vi "GetStatus.vi"(8 "error in (no error)":errorcluster, 11 "GS in":refnum<class "GuiderSetup.lvclass">) -> (0 "error out":errorcluster, 3 "GS out":refnum<class "GuiderSetup.lvclass">)   [LabVIEW 2018, in "GuiderSetup.lvclass"]
uses:
  GuiderSetup.lvclass
  C:/Users/devstaff/sparc4/s4gui/Versao ZeroMQ REQ-REP/SPARC4_GUI -v1.0.0/S4GUI/S4GUI.lvclass
  S4GUI/S4GUI.lvclass/S4GUI.ctl
  Instrument/Instrument.lvclass/Instrument.ctl
  Device/Optics/Optics.lvclass/Optics.ctl
  Server/Server.lvclass/Server.ctl
  Device/Optics/Opt_Continuous/Opt_Continuous.lvclass
  C:/Users/devstaff/sparc4/s4gui/Versao ZeroMQ REQ-REP/SPARC4_GUI -v1.0.0/Device/Optics/Optics.lvclass
  Instrument/Instrument.lvclass
  C:/Users/devstaff/sparc4/s4gui/Versao ZeroMQ REQ-REP/SPARC4_GUI -v1.0.0/Server/Server.lvclass
  S4GUI/S4GUI.lvclass
  Device/Optics/Optics.lvclass
  Server/Server.lvclass
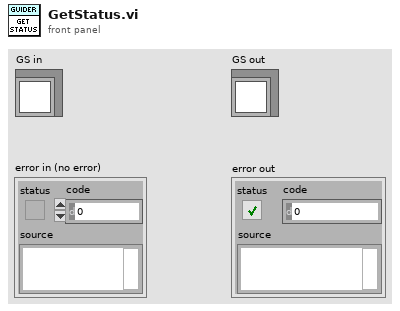
[diagram p1: front panel]
types:
  T1 = cluster{"Trigger Mode Status":string, "String output":string, "Instrument Status":cluster{"WPROT pos":dbl, "WPSEL pos":dbl, "GMIR pos":dbl, "GFOC pos":dbl, "CALW pos":dbl, "ASEL pos":dbl, "mode":bool, "String Status":string, "connection":bool, "operational":bool}, "Sync Box State":i32, "Trigger General Status":string, "Instrument States":cluster{"WPSEL State":i32, "WPROT State":i32, "CALW State":i32, "ASEL State":i32, "GMIR State":i32, "GFOC State":i32}, "Instrument Pos Names":cluster{"WPROT posname":string, "WPSEL posname":string, "CALW posname":string, "ASEL posname":string}, "ChannelA_Status":cluster{"Current exp":dbl, "Frames done":u32, "LastFileImage":string, "CamStatus":string, "Run state":u32, "connection":bool, "Cooler ON/OFF":i16, "Currently temperature":i16, "Temperature Status":string, "target  temp":i16, "conf runing":bool, "FT":bool, "UsedDisk":u16, "operational":bool}, "WPROT seq":u16, "ChannelB_Status":cluster{"Current exp":dbl, "Frames done":u32, "LastFileImage":string, "CamStatus":string, "Run state":u32, "connection":bool, "Cooler ON/OFF":i16, "Currently temperature":i16, "Temperature Status":string, "target  temp":i16, "conf runing":bool, "FT":bool, "UsedDisk":u16, "operational":bool}, "ChannelC_Status":cluster{"Current exp":dbl, "Frames done":u32, "LastFileImage":string, "CamStatus":string, "Run state":u32, "connection":bool, "Cooler ON/OFF":i16, "Currently temperature":i16, "Temperature Status":string, "target  temp":i16, "conf runing":bool, "FT":bool, "UsedDisk":u16, "operational":bool}, "ChannelD_Status":cluster{"Current exp":dbl, "Frames done":u32, "LastFileImage":string, "CamStatus":string, "Run state":u32, "connection":bool, "Cooler ON/OFF":i16, "Currently temperature":i16, "Temperature Status":string, "target  temp":i16, "conf runing":bool, "FT":bool, "UsedDisk":u16, "operational":bool}, "ChannelA_CCD":cluster{"ACQUISITION_MODE":u8, "TRIGGER_MODE":u8, "READ_MODE":u8, "PREAMP":u8, "READOUT_RATE":u8, "VERTICAL_SHIFT_SPEED":u8, "EM_MODE":u8, "EM_GAIN":u16, "SHUTTER_MODE":u8, "SHUTTER_TTL":u8, "SHUTTER_OPENNING_TIME":u16, "SHUTTER_CLOSING_TIME":u16, "VBIN":u16, "HBIN":u16, "INITIAL_LINE":u16, "INITIAL_COLUMN":u16, "FINAL_LINE":u16, "FINAL_COLUMN":u16, "FRAME_TRANSFER":bool, "VERTICAL_CLOCK_VOLTAGE":u8, "AD_CHANNEL":u32}, "ChannelB_CCD ":cluster{"ACQUISITION_MODE":u8, "TRIGGER_MODE":u8, "READ_MODE":u8, "PREAMP":u8, "READOUT_RATE":u8, "VERTICAL_SHIFT_SPEED":u8, "EM_MODE":u8, "EM_GAIN":u16, "SHUTTER_MODE":u8, "SHUTTER_TTL":u8, "SHUTTER_OPENNING_TIME":u16, "SHUTTER_CLOSING_TIME":u16, "VBIN":u16, "HBIN":u16, "INITIAL_LINE":u16, "INITIAL_COLUMN":u16, "FINAL_LINE":u16, "FINAL_COLUMN":u16, "FRAME_TRANSFER":bool, "VERTICAL_CLOCK_VOLTAGE":u8, "AD_CHANNEL":u32}, "ChannelC_CCD":cluster{"ACQUISITION_MODE":u8, "TRIGGER_MODE":u8, "READ_MODE":u8, "PREAMP":u8, "READOUT_RATE":u8, "VERTICAL_SHIFT_SPEED":u8, "EM_MODE":u8, "EM_GAIN":u16, "SHUTTER_MODE":u8, "SHUTTER_TTL":u8, "SHUTTER_OPENNING_TIME":u16, "SHUTTER_CLOSING_TIME":u16, "VBIN":u16, "HBIN":u16, "INITIAL_LINE":u16, "INITIAL_COLUMN":u16, "FINAL_LINE":u16, "FINAL_COLUMN":u16, "FRAME_TRANSFER":bool, "VERTICAL_CLOCK_VOLTAGE":u8, "AD_CHANNEL":u32}, "ChannelD_CCD":cluster{"ACQUISITION_MODE":u8, "TRIGGER_MODE":u8, "READ_MODE":u8, "PREAMP":u8, "READOUT_RATE":u8, "VERTICAL_SHIFT_SPEED":u8, "EM_MODE":u8, "EM_GAIN":u16, "SHUTTER_MODE":u8, "SHUTTER_TTL":u8, "SHUTTER_OPENNING_TIME":u16, "SHUTTER_CLOSING_TIME":u16, "VBIN":u16, "HBIN":u16, "INITIAL_LINE":u16, "INITIAL_COLUMN":u16, "FINAL_LINE":u16, "FINAL_COLUMN":u16, "FRAME_TRANSFER":bool, "VERTICAL_CLOCK_VOLTAGE":u8, "AD_CHANNEL":u32}, "CHA_Checked Params":cluster{"ACQUISITION_MODE":bool, "TRIGGER_MODE":bool, "READ_MODE":bool, "PREAMP":bool, "READOUT_RATE":bool, "VERTICAL_SHIFT_SPEED":bool, "EM_MODE":bool, "EM_GAIN":bool, "SHUTTER_MODE":bool, "SHUTTER_TTL":bool, "SHUTTER_OPENING_TIME":bool, "SHUTTER_CLOSING_TIME":bool, "VBIN":bool, "HBIN":bool, "INITIAL_LINE":bool, "INITIAL_COLUMN":bool, "FINAL_LINE":bool, "FINAL_COLUMN":bool, "FRAME_TRANSFER":bool, "VERTICAL_CLOCK_VOLTAGE":bool, "AD_CHANNEL":bool}, "CHB_Checked Params":cluster{"ACQUISITION_MODE":bool, "TRIGGER_MODE":bool, "READ_MODE":bool, "PREAMP":bool, "READOUT_RATE":bool, "VERTICAL_SHIFT_SPEED":bool, "EM_MODE":bool, "EM_GAIN":bool, "SHUTTER_MODE":bool, "SHUTTER_TTL":bool, "SHUTTER_OPENING_TIME":bool, "SHUTTER_CLOSING_TIME":bool, "VBIN":bool, "HBIN":bool, "INITIAL_LINE":bool, "INITIAL_COLUMN":bool, "FINAL_LINE":bool, "FINAL_COLUMN":bool, "FRAME_TRANSFER":bool, "VERTICAL_CLOCK_VOLTAGE":bool, "AD_CHANNEL":bool}, "CHC_Checked Params":cluster{"ACQUISITION_MODE":bool, "TRIGGER_MODE":bool, "READ_MODE":bool, "PREAMP":bool, "READOUT_RATE":bool, "VERTICAL_SHIFT_SPEED":bool, "EM_MODE":bool, "EM_GAIN":bool, "SHUTTER_MODE":bool, "SHUTTER_TTL":bool, "SHUTTER_OPENING_TIME":bool, "SHUTTER_CLOSING_TIME":bool, "VBIN":bool, "HBIN":bool, "INITIAL_LINE":bool, "INITIAL_COLUMN":bool, "FINAL_LINE":bool, "FINAL_COLUMN":bool, "FRAME_TRANSFER":bool, "VERTICAL_CLOCK_VOLTAGE":bool, "AD_CHANNEL":bool}, "CHD_Checked Params":cluster{"ACQUISITION_MODE":bool, "TRIGGER_MODE":bool, "READ_MODE":bool, "PREAMP":bool, "READOUT_RATE":bool, "VERTICAL_SHIFT_SPEED":bool, "EM_MODE":bool, "EM_GAIN":bool, "SHUTTER_MODE":bool, "SHUTTER_TTL":bool, "SHUTTER_OPENING_TIME":bool, "SHUTTER_CLOSING_TIME":bool, "VBIN":bool, "HBIN":bool, "INITIAL_LINE":bool, "INITIAL_COLUMN":bool, "FINAL_LINE":bool, "FINAL_COLUMN":bool, "FRAME_TRANSFER":bool, "VERTICAL_CLOCK_VOLTAGE":bool, "AD_CHANNEL":bool}, "Trigger_connection":bool, "TCSPD_connection":bool, "TCS extended":string, "TCS id":u32, "S4ICS id":u32, "focus pos":i32, "Focus_connection":bool, "WS_connection":bool, "weather status":cluster{"broker":string, "version":string, "date":string, "hour":string, "outHumidity":string, "inHumidity":string, "inTemp":string, "outTemp":string, "windSpeed":string, "windDirection":string, "pressure":string, "dewOut":string, "dewIn":string, "leaf":string, "rain":string, "windChill":string}, "GS STATUS cluster":cluster{"FocusPhot":dbl, "FocusPolar":dbl, "FocusEffic":dbl, "FocusInstrum":dbl, "ICS":bool, "AG":bool, "BROKER":string}, "TCSPD_operational":bool, "Focus_operational":bool}
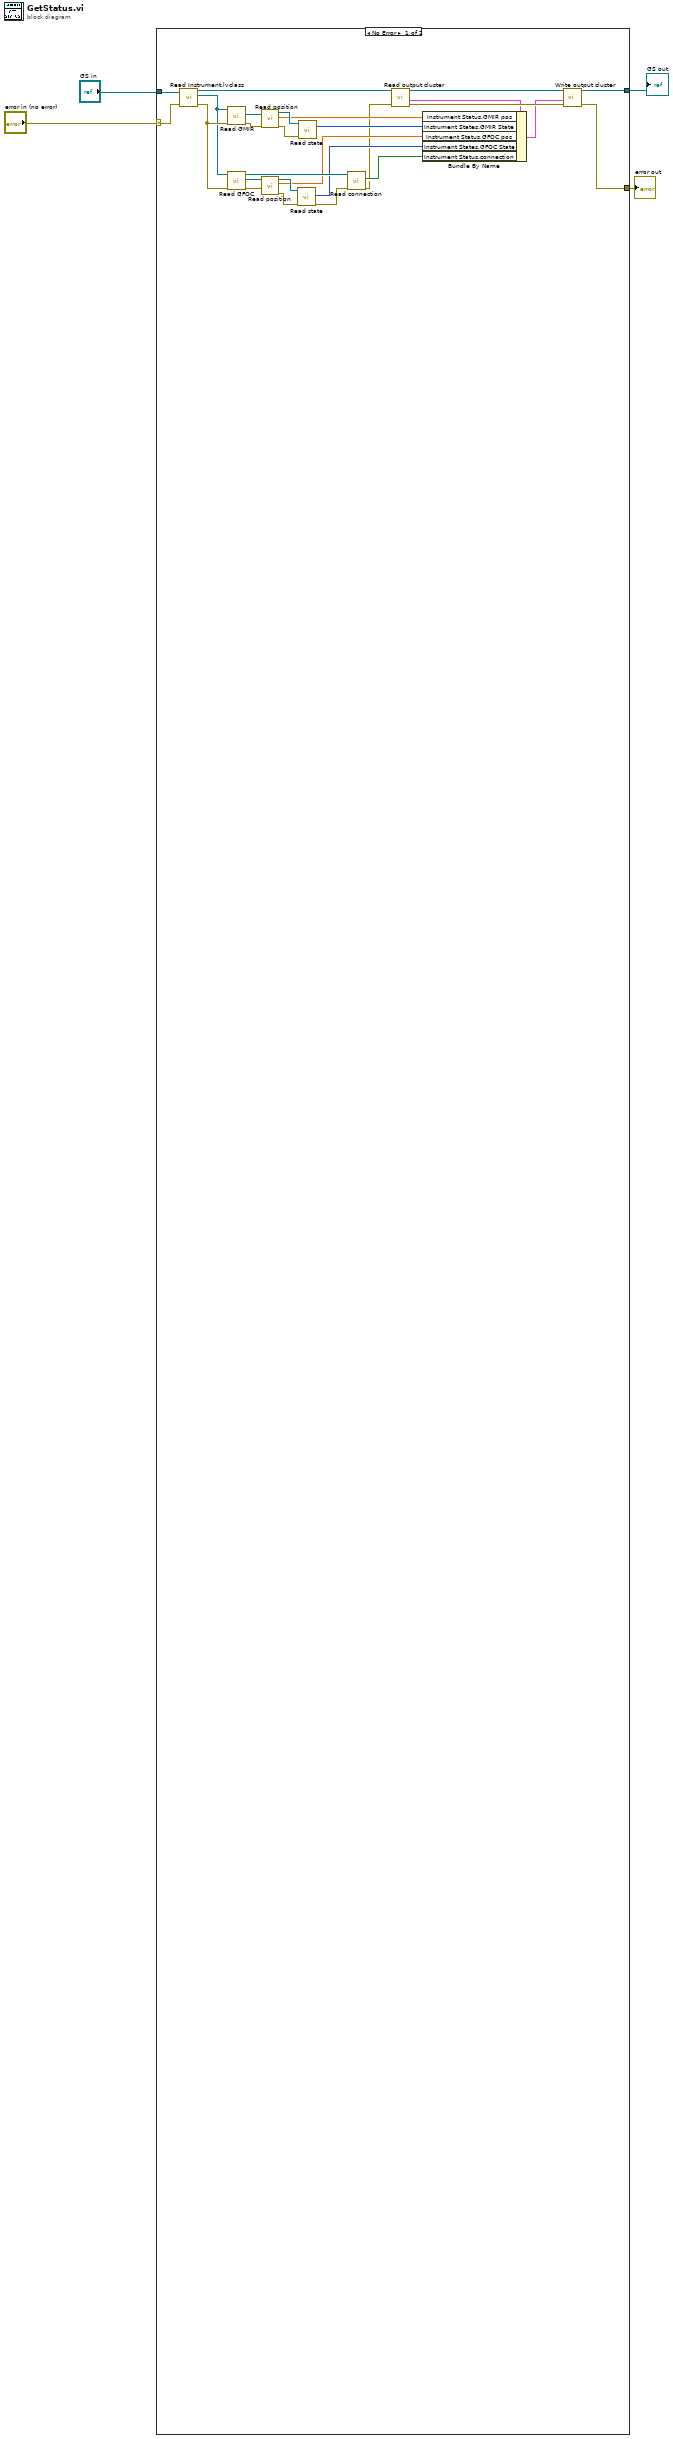
[diagram p0: block diagram]
diagram:
  n1 = case shown="No Error" "error in (no error)" {
    selector: "error in (no error)" -> [w20 w32]
    tunnel: "GS in" -> [w19 w33]
    tunnel: [w12 w33] -> w2
    tunnel: [w11 w32] -> w1
    frame No Error {
      n2 = call "Read Instrument.lvclass.vi"("error in (no error)"=w20, "S4ACS_GUI in"=w19) -> ("error out"=w21:errorcluster, "Instrument.lvclass"=w18:refnum<class "Instrument.lvclass">, "S4ACS_GUI out"=w10:refnum<class "GuiderSetup.lvclass">)  [unwired: 7 in]
      n3 = call "Read GMIR.vi"("error in (no error)"=w21, "Instrument in"=w18) -> ("error out"=w31:errorcluster, "Opt_Continuous.lvclass"=w30:refnum<class "Opt_Continuous.lvclass">)  [unwired: 7 in, 1 out]
      n4 = call "Read GFOC.vi"("error in (no error)"=w21, "Instrument in"=w18) -> ("error out"=w28:errorcluster, "Opt_Continuous.lvclass"=w29:refnum<class "Opt_Continuous.lvclass">, "Instrument out"=w23:refnum<class "Instrument.lvclass">)  [unwired: 7 in]
      n5 = call "Read position.vi"("error in (no error)"=w31, "Optics in"=w30) -> ("error out"=w26:errorcluster, "position"=w16:dbl, "Optics out"=w27:refnum<class "Opt_Continuous.lvclass">)  [unwired: 7 in]
      n6 = call "Read position.vi"("error in (no error)"=w28, "Optics in"=w29) -> ("error out"=w24:errorcluster, "position"=w14:dbl, "Optics out"=w25:refnum<class "Opt_Continuous.lvclass">)  [unwired: 7 in]
      n7 = call-dynamic "Read state.vi"("error in (no error)"=w24, "Optics in"=w25) -> ("error out"=w22:errorcluster, "state"=w13:u8)  [unwired: 7 in, 1 out]
      n8 = call-dynamic "Read state.vi"("error in (no error)"=w26, "Optics in"=w27) -> ("state"=w15:u8)  [unwired: 7 in, 2 out]
      n9 = call "Read connection.vi"("error in (no error)"=w22, "Server in"=w23) -> ("error out"=w8:errorcluster, "connection"=w17:bool)  [unwired: 7 in, 1 out]
      n10 = call-dynamic "Read output cluster.vi"("error in (no error)"=w8, "S4GUI in"=w10) -> ("error out"=w7:errorcluster, "output cluster"=w6:T1, "S4GUI out"=w9:refnum<class "GuiderSetup.lvclass">)  [unwired: 7 in]
      n11 = Bundle By Name(cluster=w6, "Instrument Status.GMIR pos"=w16, "Instrument States.GMIR State"=w15, "Instrument Status.GFOC pos"=w14, "Instrument States.GFOC State"=w13, "Instrument Status.connection"=w17) -> (w5:T1)
      n12 = call-dynamic "Write output cluster.vi"("error in (no error)"=w7, "output cluster"=w5, "S4GUI in"=w9) -> ("error out"=w11:errorcluster, "S4GUI out"=w12:refnum<class "GuiderSetup.lvclass">)  [unwired: 7 in]
    }
    frame Error {
    }
  }
  "GS out" <- w2
  "error out" <- w1
